vi "PressureGaugeWithSmallWindow.vi"(4 "Error In":errorcluster, 7 "Command":string) -> (0 "Error Out":errorcluster, 3 "Response":string)   [LabVIEW 2018]
uses:
  MOKO_LabViewLibrary/MokoLowLevel/MokoLowLovelControl/MLLC_Mode.ctl
  data/PressureGaugeInfo_1.ctl
panel:
  in  "Utility name":string="PRESSURESTORE"
  in  "Error Code":i32=5475
  in  "UtilitySettings":T2={"Permanent data"={"Информация об образце"={"Тип"="Манометр", "Владелец"="Компания \"MOKO\"", "Номер клейма"="111222", "Пределы допускаемой погрешности "=0.05, "Производственный № прибора"="111222333", "Наименование СИ"="Манометр"}, "Информация о поверке"={"Место проведения поверки"="Планета земля", "Поверку провел"="Johnny Respect", "Номер заказа"="1", "Номер рабочего места"="1", "ДД"=21.0, "ММ"="Январь", "ГГГГ"=2022.0, "№ протокола"="G-111111", "№ манометра"=5555.0}, "Характеристики манометра"={"Максимум шкалы"=10.0, "1-ая точка"=2.0, "Единица измерения"="МПа", "Цена деления"=2.0, "Класс точности"="0,4", "Минимум шкалы"=2.0, "Количество точек"=0.0}, "Условия поверки"={"Температура воздуха"=22.0, "Влажность воздуха"=60.0, "Давление"=750.0}, "Драйвер"="Simulation", "Поверяемая точка"=0.0}, "Saved Data"=variant(cluster{"Информация об образце":cluster{"Тип":string, "Владелец":string, "Номер клейма":string, "Пределы допускаемой погрешности ":dbl, "Производственный № прибора":string, "Наименование СИ":string}, "Информация о поверке":cluster{"Место проведения поверки":string, "Поверку провел":string, "Номер заказа":string, "Номер рабочего места":string, "ДД":dbl, "ММ":string, "ГГГГ":dbl, "№ протокола":string, "№ манометра":dbl}, "Характеристики манометра":cluster{"Максимум шкалы":dbl, "1-ая точка":dbl, "Единица измерения":string, "Цена деления":dbl, "Класс точности":string, "Минимум шкалы":dbl, "Количество точек":dbl}, "Условия поверки":cluster{"Температура воздуха":dbl, "Влажность воздуха":dbl, "Давление":dbl}, "Драйвер":string, "Поверяемая точка":dbl} {"Информация об образце"={"Тип"="Манометр", "Владелец"="Компания \"MOKO\"", "Номер клейма"="111222333", "Пределы допускаемой погрешности "=0.05, "Производственный № прибора"="111222333", "Наименование СИ"="Манометр"}, "Информация о поверке"={"Место проведения поверки"="Планета земля", "Поверку провел"="Johnny Respect", "Номер заказа"="1", "Номер рабочего места"="1", "ДД"=21.0, "ММ"="Январь", "ГГГГ"=2022.0, "№ протокола"="G-111111", "№ манометра"=1123123.0}, "Характеристики манометра"={"Максимум шкалы"=10.0, "1-ая точка"=2.0, "Единица измерения"="МПа", "Цена деления"=2.0, "Класс точности"="0,4", "Минимум шкалы"=2.0, "Количество точек"=0.0}, "Условия поверки"={"Температура воздуха"=22.0, "Влажность воздуха"=60.0, "Давление"=750.0}, "Драйвер"="Simulation", "Поверяемая точка"=0.0}), "waittime"=30000.0, "BAD"=0.0, "Defect"=FALSE}
  in  "Mode":T3=enum."Check"
  # "PressureGauge"
  # "Default Settings"
  # "Temporary data"
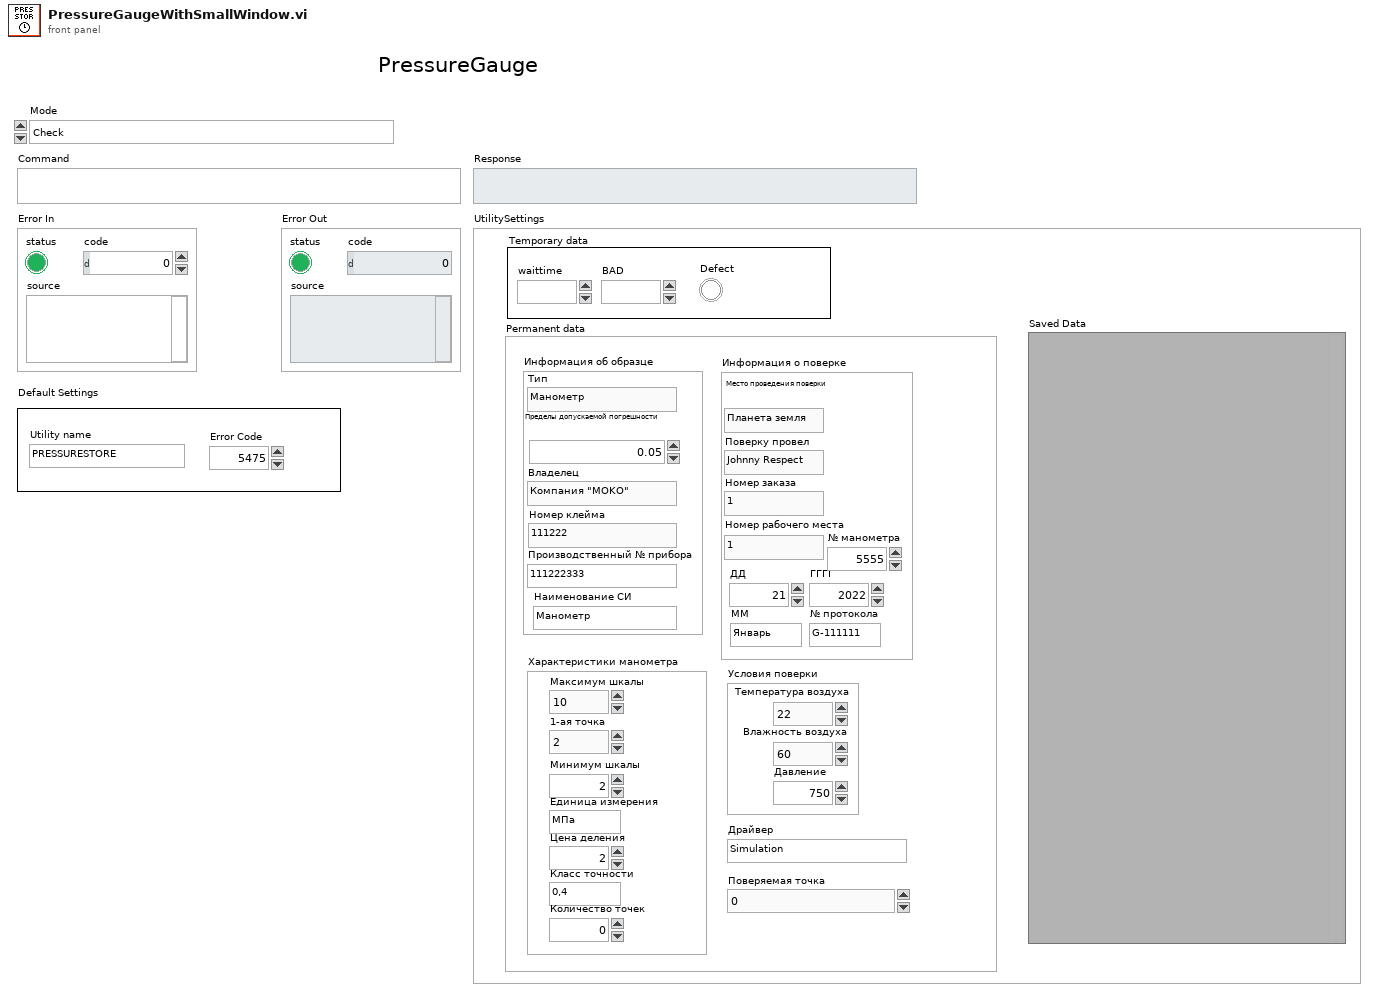
[diagram p1: front panel]
types:
  T1 = typedef "PressureGaugeInfo_1.ctl" = cluster{"Информация об образце":cluster{"Тип":string, "Владелец":string, "Номер клейма":string, "Пределы допускаемой погрешности ":dbl, "Производственный № прибора":string, "Наименование СИ":string}, "Информация о поверке":cluster{"Место проведения поверки":string, "Поверку провел":string, "Номер заказа":string, "Номер рабочего места":string, "ДД":dbl, "ММ":string, "ГГГГ":dbl, "№ протокола":string, "№ манометра":dbl}, "Характеристики манометра":cluster{"Максимум шкалы":dbl, "1-ая точка":dbl, "Единица измерения":string, "Цена деления":dbl, "Класс точности":string, "Минимум шкалы":dbl, "Количество точек":dbl}, "Условия поверки":cluster{"Температура воздуха":dbl, "Влажность воздуха":dbl, "Давление":dbl}, "Драйвер":string, "Поверяемая точка":dbl}
  T2 = cluster{"Permanent data":T1, "Saved Data":variant, "waittime":dbl, "BAD":dbl, "Defect":bool}
  T3 = typedef "MLLC_Mode.ctl" = enum16{"get", "set", "close", "Init", "Check"}
  T4 = typedef "MLLC_Error.ctl" = errorcluster
  T5 = typedef "PressureGaugeInfo.ctl" = cluster{"Информация об образце":cluster{"Тип":string, "Владелец":string, "Номер клейма":string, "Пределы допускаемой погрешности ":dbl, "Производственный № прибора":string, "Наименование СИ":string}, "Информация о поверке":cluster{"Место проведения поверки":string, "Поверку провел":string, "Номер заказа":string, "Номер рабочего места":string, "ДД":dbl, "ММ":string, "ГГГГ":dbl, "№ протокола":string, "№ манометра":dbl}, "Характеристики манометра":cluster{"Максимум шкалы":dbl, "1-ая точка":dbl, "Единица измерения":string, "Цена деления":dbl, "Класс точности":string, "Минимум шкалы":dbl, "Количество точек":dbl}, "Условия поверки":cluster{"Температура воздуха":dbl, "Влажность воздуха":dbl, "Давление":dbl}, "Драйвер":string, "Поверяемая точка":dbl}
  T6 = typedef "MLLC_Command.ctl" = string
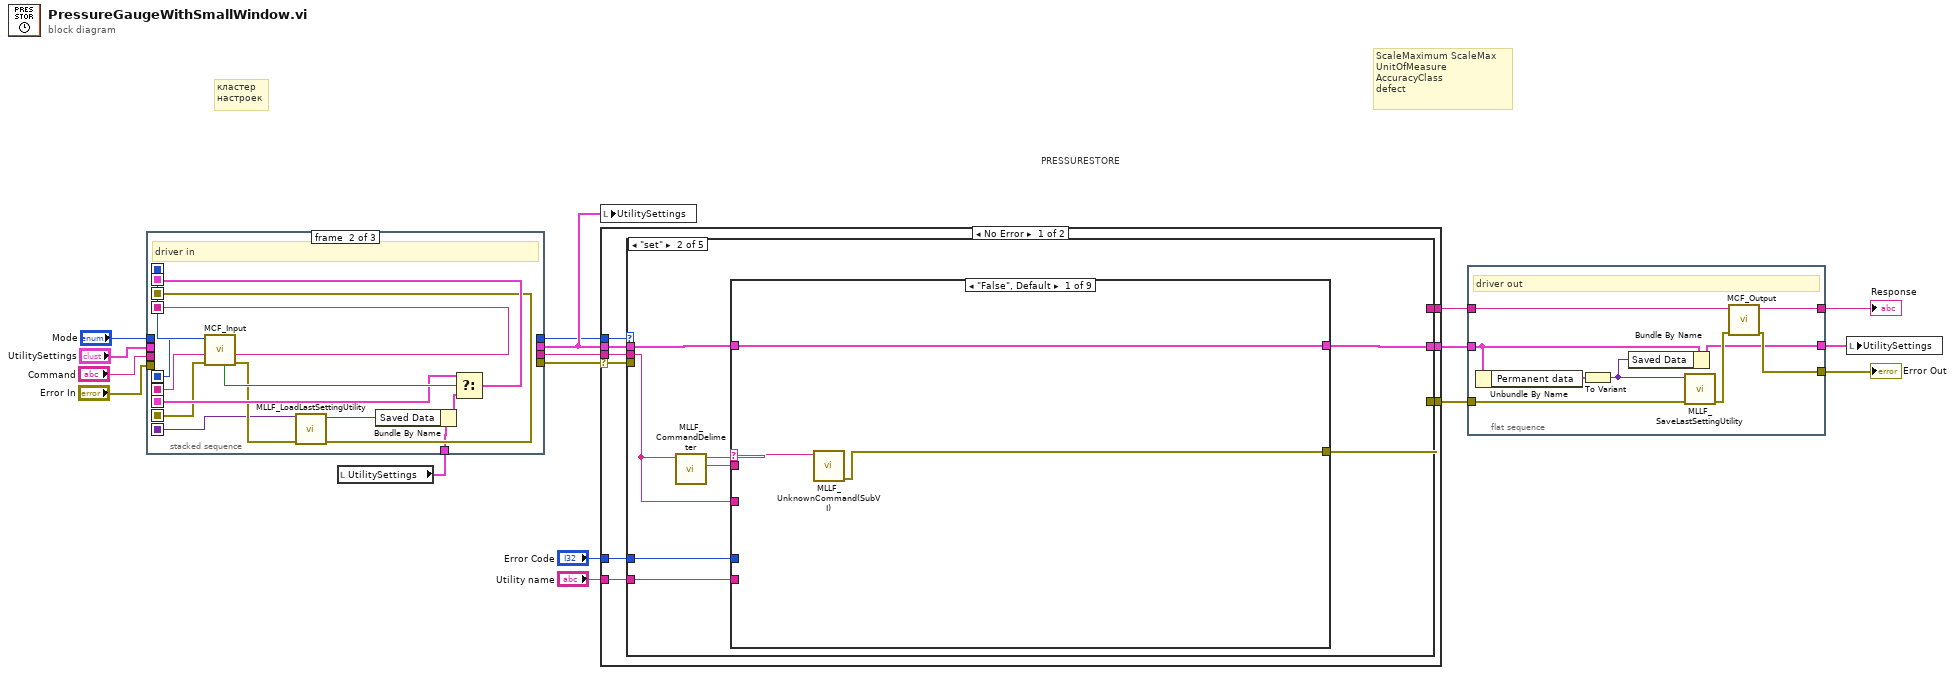
[diagram p0: block diagram]
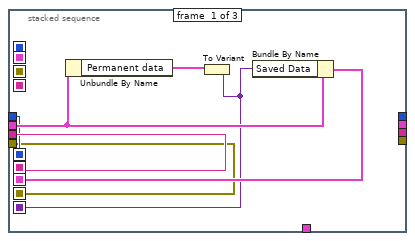
[diagram p2: hidden frame]
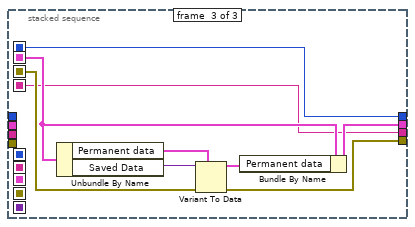
[diagram p3: hidden frame]
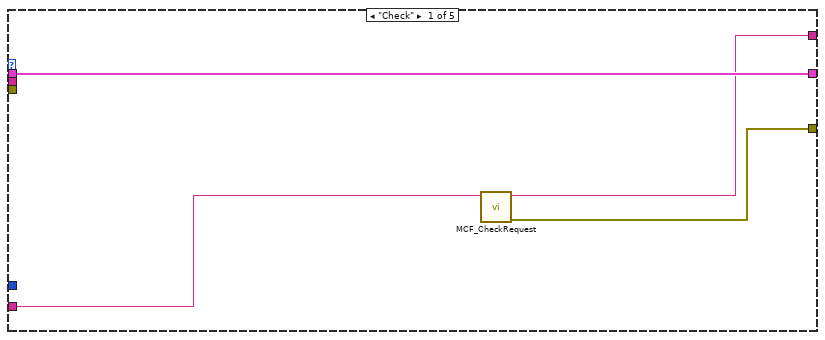
[diagram p4: hidden frame]
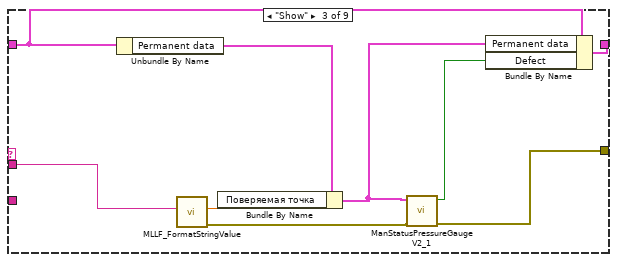
[diagram p6: hidden frame]
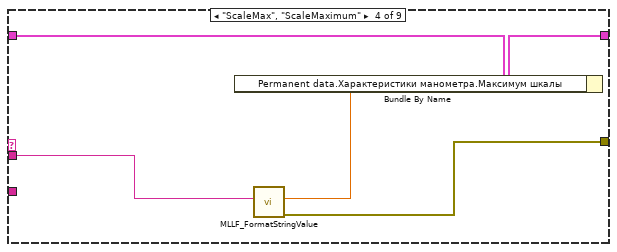
[diagram p7: hidden frame]
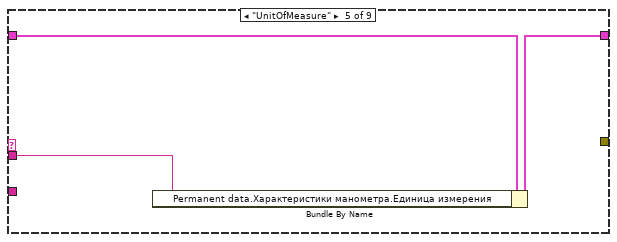
[diagram p8: hidden frame]
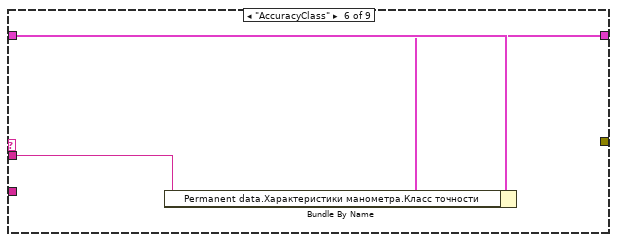
[diagram p9: hidden frame]
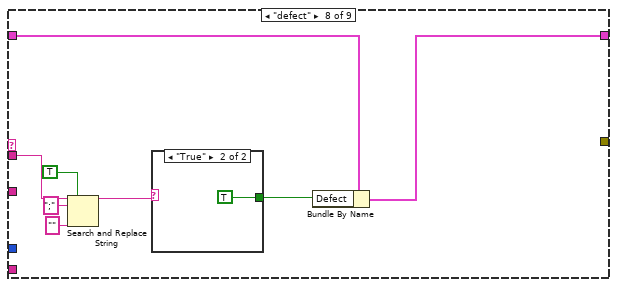
[diagram p11: hidden frame]
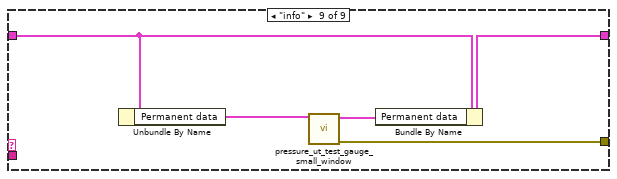
[diagram p13: hidden frame]
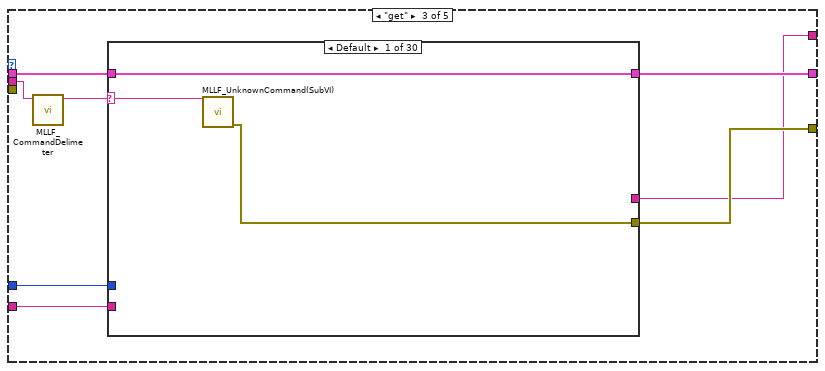
[diagram p14: hidden frame]
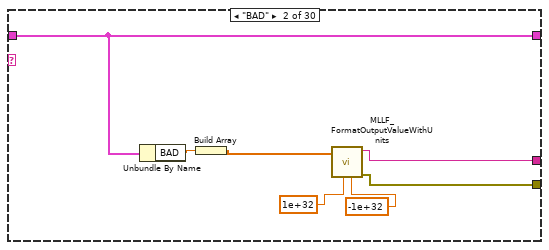
[diagram p15: hidden frame]
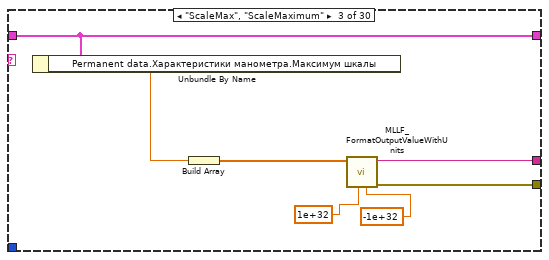
[diagram p16: hidden frame]
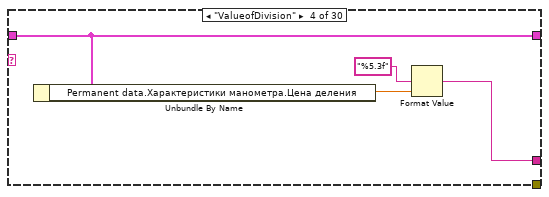
[diagram p17: hidden frame]
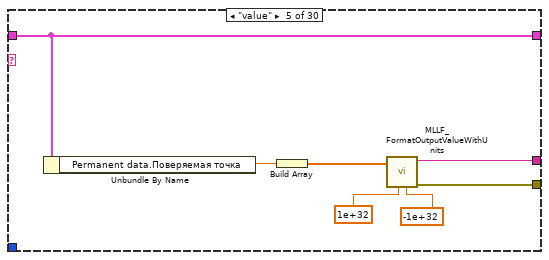
[diagram p18: hidden frame]
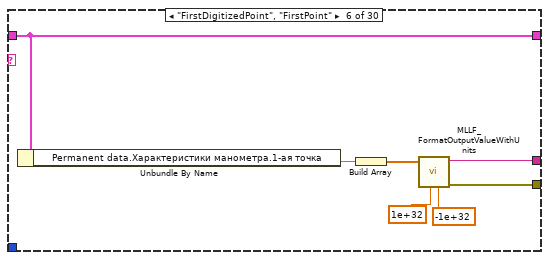
[diagram p19: hidden frame]
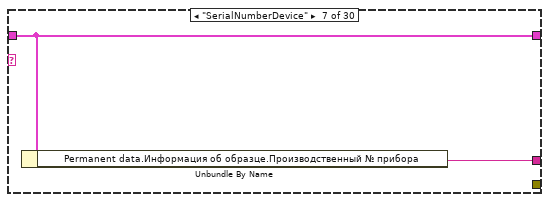
[diagram p20: hidden frame]
diagram:
  # "ScaleMaximum ScaleMax\nUnitOfMeasure\nAccuracyClass\ndefect"
  # "кластер\nнастроек"
  # "PRESSURESTORE"
  n1 = local read "UtilitySettings"() -> (w12:T2)
  n2 = stacked-sequence {
    seq-local: [w20 _ _] -> [_ w36 _]
    seq-local: [w19 _ _] -> [_ w37 _]
    seq-local: [w22 _ _] -> [_ w32 _]
    seq-local: [w18 _ _] -> [_ w31 _]
    seq-local: [w21 _ _] -> [_ w26 _]
    seq-local: [_ w27 _] -> [_ _ w43]
    seq-local: [_ w38 _] -> [_ _ w40]
    seq-local: [_ w35 _] -> [_ _ w39]
    seq-local: [_ w34 _] -> [_ _ w44]
    tunnel: "Command" -> [w20 _ _]
    tunnel: "Mode" -> [w19 _ _]
    tunnel: "Error In" -> [w18 _ _]
    tunnel: "UtilitySettings" -> [w23 _ _]
    tunnel: w12 -> [_ w25 _]
    tunnel: [_ _ w39] -> w8
    tunnel: [_ _ w42] -> w11
    tunnel: [_ _ w41] -> w10
    tunnel: [_ _ w40] -> w9
    frame #0 {
      n3 = Unbundle By Name(w23) -> ("Permanent data"=w24:T1)
      n4 = To Variant(anything=w24) -> (Variant=w21:variant)
      n5 = Bundle By Name(cluster=w23, "Saved Data"=w21) -> (w22:T2)
    }
    frame #1 {
      # "driver in"
      n6 = call "MCF_Input.vi"("error in (no error)"=w31, "Command"=w36, "Mode"=w37) -> ("error out"=w30:errorcluster, "Command out"=w35:string, "Mode out"=w38:T3, "Boolean"=w33:bool)  [unwired: 5 in]
      n7 = call "MLLF_LoadLastSettingUtility.vi"("Error In"=w30, "Save data in"=w26) -> ("Error Out"=w27:errorcluster, "Save data out"=w29:variant)  [unwired: 8 in]
      n8 = Bundle By Name(cluster=w25, "Saved Data"=w29) -> (w28:T2)
      n9 = Select(t=w32, s=w33, f=w28) -> (s? t:f=w34:T2)
    }
    frame #2 {
      n10 = Unbundle By Name(w44) -> ("Permanent data"=w45:T1, "Saved Data"=w47:variant)
      n11 = Variant To Data(error in=w43, type=w45, Variant=w47) -> (data=w46:T1, error out=w41:errorcluster)
      n12 = Bundle By Name(cluster=w44, "Permanent data"=w46) -> (w42:T2)
    }
  }
  n13 = local write "UtilitySettings"(w11) -> ()
  n14 = case shown="No Error" w10 {
    selector: w10 -> [w52 w234]
    tunnel: [w54 w234] -> w16
    tunnel: w9 -> [w56 _]
    tunnel: [w55 _] -> w14
    tunnel: w8 -> [w53 _]
    tunnel: w11 -> [w49 w233]
    tunnel: "Error Code" -> [w51 _]
    tunnel: "Utility name" -> [w50 _]
    tunnel: [w48 w233] -> w15
    frame No Error {
      n15 = case shown="\"set\"" w56 {
        tunnel: [w58 _ w108 _ _] -> w55
        tunnel: [w57 w68 w109 _ _] -> w54
        tunnel: w53 -> [_ w63 w115 _ _]
        tunnel: w52 -> [_ _ _ _ _]
        tunnel: w51 -> [_ w67 w112 _ _]
        tunnel: w50 -> [w59 w64 w111 _ _]
        tunnel: w49 -> [w60 w66 w114 w231 w232]
        tunnel: [w60 w65 w113 w231 w232] -> w48
        frame "Check" {
          n16 = call "MCF_CheckRequest.vi"("Driver Name"=w59) -> ("Error Out"=w57:errorcluster, "Output String"=w58:string)  [unwired: 9 in]
        }
        frame "set" {
          n17 = call "MLLF_CommandDelimeter.vi"("command with param"=w63) -> ("param 1"=w61:string, "command"=w62:string)  [unwired: 7 in, 2 out]
          n18 = case shown="\"False\", Default" w62 {
            selector: w62 -> [w70 _ _ _ _ _ _ _ _]
            tunnel: w61 -> [_ _ w78 w82 w88 w92 _ w99 _]
            tunnel: w63 -> [_ _ _ _ _ _ _ _ _]
            tunnel: [w69 _ w75 w86 _ _ _ _ w107] -> w68
            tunnel: w67 -> [_ _ _ _ _ _ _ _ _]
            tunnel: w66 -> [w71 w72 w80 w84 w89 w91 w93 w101 w106]
            tunnel: [w71 w72 w79 w83 w87 w90 w93 w100 w105] -> w65
            tunnel: w64 -> [_ _ _ _ _ _ _ _ _]
            frame "False", Default {
              n19 = call "MLLF_UnknownCommand(SubVI).vi"("Unknown command"=w70) -> ("error out"=w69:errorcluster)  [unwired: 10 in]
            }
            frame "<----MAIN FUNCTIONS---->" {
            }
            frame "Show" {
              n20 = Unbundle By Name(w80) -> ("Permanent data"=w74:T1)
              n21 = call "MLLF_FormatStringValue.vi"("String Value"=w78) -> ("error out"=w77:T4, "number"=w81:dbl)  [unwired: 8 in, 1 out]
              n22 = Bundle By Name(cluster=w74, "Поверяемая точка"=w81) -> (w73:T1)
              n23 = call "ManStatusPressureGaugeV2_1.vi"("Error In"=w77, "Show in"=w73) -> ("Error Out"=w75:errorcluster, "defect"=w76:bool)  [unwired: 8 in]
              n24 = Bundle By Name(cluster=w80, "Permanent data"=w73, "Defect"=w76) -> (w79:T2)
            }
            frame "ScaleMax", "ScaleMaximum" {
              n25 = call "MLLF_FormatStringValue.vi"("String Value"=w82) -> ("error out"=w86:T4, "number"=w85:dbl)  [unwired: 8 in, 1 out]
              n26 = Bundle By Name(cluster=w84, "Permanent data.Характеристики манометра.Максимум шкалы"=w85) -> (w83:T2)
            }
            frame "UnitOfMeasure" {
              n27 = Bundle By Name(cluster=w89, "Permanent data.Характеристики манометра.Единица измерения"=w88) -> (w87:T2)
            }
            frame "AccuracyClass" {
              n28 = Bundle By Name(cluster=w91, "Permanent data.Характеристики манометра.Класс точности"=w92) -> (w90:T2)
            }
            frame "---------ADDITIONAL---------" {
            }
            frame "defect" {
              n29 = Search and Replace String(replace all?=TRUE ("replace all? (F)"), input string=w99, search string=";", replace string="" ("replace string (\"\")")) -> (result string=w95:string)  [unwired: 4 in, 3 out]
              n30 = case shown="\"True\"" w95 {
                tunnel: [_ TRUE] -> w94
                frame "False", Default {
                }
                frame "True" {
                }
              }
              n31 = Bundle By Name(cluster=w101, "Defect"=w94) -> (w100:T2)
            }
            frame "info" {
              n32 = Unbundle By Name(w106) -> ("Permanent data"=w103:T1)
              n33 = call "pressure_ut_test_gauge_small_window.vi"("Manometr in"=w103) -> ("Error Out"=w107:errorcluster, "Manometr out"=w104:T5)  [unwired: 9 in]
              n34 = Bundle By Name(cluster=w106, "Permanent data"=w104) -> (w105:T2)
            }
          }
        }
        frame "get" {
          n35 = call "MLLF_CommandDelimeter.vi"("command with param"=w115) -> ("command"=w110:string)  [unwired: 7 in, 3 out]
          n36 = case shown="Default" w110 {
            selector: w110 -> [w117 _ _ _ _ _ _ _ _ _ _ _ _ _ _ _ _ _ _ _ _ _ _ _ _ _ _ _ _ _]
            tunnel: w112 -> [_ _ _ _ _ _ _ _ _ _ _ _ _ _ _ _ _ _ _ _ _ _ _ _ _ _ _ _ _ _]
            tunnel: [w118 w125 w132 w136 w143 w150 w152 w154 w161 w168 w170 w172 w174 w181 w183 w186 w188 w191 w193 w197 w199 w203 w205 w209 w211 w215 w219 w223 w225 w230] -> w113
            tunnel: w114 -> [w118 w125 w132 w136 w143 w150 w152 w154 w161 w168 w170 w172 w174 w181 w183 w186 w188 w191 w193 w197 w199 w203 w205 w209 w211 w215 w219 w223 w225 w230]
            tunnel: w111 -> [_ _ _ _ _ _ _ _ _ _ _ _ _ _ _ _ _ _ _ _ _ _ _ _ _ _ _ _ _ _]
            tunnel: [w116 w120 w126 _ w138 w145 _ _ w155 w162 _ _ _ w175 _ _ _ _ _ _ _ _ _ _ _ _ _ _ _ _] -> w109
            tunnel: [_ w121 w127 w133 w137 w146 w151 w153 w156 w163 w169 w171 w173 w176 w182 w184 w187 w189 w192 w194 w198 w200 w204 w206 w210 w212 w216 w220 w224 w226] -> w108
            frame Default {
              n37 = call "MLLF_UnknownCommand(SubVI).vi"("Unknown command"=w117) -> ("error out"=w116:errorcluster)  [unwired: 10 in]
            }
            frame "BAD" {
              n38 = Unbundle By Name(w125) -> ("BAD"=w124:dbl)
              n39 = Build Array(w124) -> (w122:dbl[])
              n40 = call "MLLF_FormatOutputValueWithUnits.vi"("Lower limit"=-1e+32, "Upper limit"=1e+32, "ValuesIn"=w122) -> ("error out"=w120:T4, "Result string"=w121:T6)  [unwired: 7 in]
            }
            frame "ScaleMax", "ScaleMaximum" {
              n41 = Unbundle By Name(w132) -> ("Permanent data.Характеристики манометра.Максимум шкалы"=w131:dbl)
              n42 = Build Array(w131) -> (w128:dbl[])
              n43 = call "MLLF_FormatOutputValueWithUnits.vi"("Lower limit"=-1e+32, "Upper limit"=1e+32, "ValuesIn"=w128) -> ("error out"=w126:T4, "Result string"=w127:T6)  [unwired: 7 in]
            }
            frame "ValueofDivision" {
              n44 = Unbundle By Name(w136) -> ("Permanent data.Характеристики манометра.Цена деления"=w134:dbl)
              n45 = Format Value(format string="%5.3f", value (0)=w134) -> (output string=w133:string)  [unwired: 1 in]
            }
            frame "value" {
              n46 = Unbundle By Name(w143) -> ("Permanent data.Поверяемая точка"=w142:dbl)
              n47 = Build Array(w142) -> (w139:dbl[])
              n48 = call "MLLF_FormatOutputValueWithUnits.vi"("Lower limit"=-1e+32, "Upper limit"=1e+32, "ValuesIn"=w139) -> ("error out"=w138:T4, "Result string"=w137:T6)  [unwired: 7 in]
            }
            frame "FirstDigitizedPoint", "FirstPoint" {
              n49 = Unbundle By Name(w150) -> ("Permanent data.Характеристики манометра.1-ая точка"=w149:dbl)
              n50 = Build Array(w149) -> (w147:dbl[])
              n51 = call "MLLF_FormatOutputValueWithUnits.vi"("Lower limit"=-1e+32, "Upper limit"=1e+32, "ValuesIn"=w147) -> ("error out"=w145:T4, "Result string"=w146:T6)  [unwired: 7 in]
            }
            frame "SerialNumberDevice" {
              n52 = Unbundle By Name(w152) -> ("Permanent data.Информация об образце.Производственный № прибора"=w151:string)
            }
            frame "NameMI" {
              n53 = Unbundle By Name(w154) -> ("Permanent data.Информация об образце.Наименование СИ"=w153:string)
            }
            frame "NumOfPoints" {
              n54 = Unbundle By Name(w161) -> ("Permanent data.Характеристики манометра.Количество точек"=w160:dbl)
              n55 = Build Array(w160) -> (w157:dbl[])
              n56 = call "MLLF_FormatOutputValueWithUnits.vi"("Lower limit"=-1e+32, "Upper limit"=1e+32, "ValuesIn"=w157) -> ("error out"=w155:T4, "Result string"=w156:T6)  [unwired: 7 in]
            }
            frame "ScaleMin" {
              n57 = Unbundle By Name(w168) -> ("Permanent data.Характеристики манометра.Минимум шкалы"=w167:dbl)
              n58 = Build Array(w167) -> (w164:dbl[])
              n59 = call "MLLF_FormatOutputValueWithUnits.vi"("Lower limit"=-1e+32, "Upper limit"=1e+32, "ValuesIn"=w164) -> ("error out"=w162:T4, "Result string"=w163:T6)  [unwired: 7 in]
            }
            frame "UnitOfMeasure" {
              n60 = Unbundle By Name(w170) -> ("Permanent data.Характеристики манометра.Единица измерения"=w169:string)
            }
            frame "AccuracyClass" {
              n61 = Unbundle By Name(w172) -> ("Permanent data.Характеристики манометра.Класс точности"=w171:string)
            }
            frame "TypeofUnit" {
              n62 = Unbundle By Name(w174) -> ("Permanent data.Информация об образце.Тип"=w173:string)
            }
            frame "PermissibleError" {
              (unwired) "%5.4f" ("format string")
              n63 = Unbundle By Name(w181) -> ("Permanent data.Информация об образце.Пределы допускаемой погрешности"=w180:dbl)
              n64 = Build Array(w180) -> (w177:dbl[])
              n65 = call "MLLF_FormatOutputValueWithUnits.vi"("Lower limit"=-1e+32, "Upper limit"=1e+32, "ValuesIn"=w177) -> ("error out"=w175:T4, "Result string"=w176:T6)  [unwired: 7 in]
            }
            frame "StampNumber" {
              n66 = Unbundle By Name(w183) -> ("Permanent data.Информация об образце.Номер клейма"=w182:string)
            }
            frame "Owner" {
              n67 = Unbundle By Name(w186) -> ("Permanent data.Информация об образце.Владелец"=w185:string)
              n68 = call "MLLF_ReplaceTwoQuotesWithOne.vi"("String in"=w185) -> ("Result string"=w184:string)  [unwired: 7 in, 3 out]
            }
            frame "Verifier" {
              n69 = Unbundle By Name(w188) -> ("Permanent data.Информация о поверке.Поверку провел"=w187:string)
            }
            frame "VerificationLocation" {
              n70 = Unbundle By Name(w191) -> ("Permanent data.Информация о поверке.Место проведения поверки"=w190:string)
              n71 = call "MLLF_ReplaceTwoQuotesWithOne.vi"("String in"=w190) -> ("Result string"=w189:string)  [unwired: 7 in, 3 out]
            }
            frame "WorkplaceNumber" {
              n72 = Unbundle By Name(w193) -> ("Permanent data.Информация о поверке.Номер рабочего места"=w192:string)
            }
            frame "UnitNumber" {
              n73 = Unbundle By Name(w197) -> ("Permanent data.Информация о поверке.№ манометра"=w195:dbl)
              n74 = Format Value(format string="%5.1f", value (0)=w195) -> (output string=w194:string)  [unwired: 1 in]
            }
            frame "OrderNumber" {
              n75 = Unbundle By Name(w199) -> ("Permanent data.Информация о поверке.Номер заказа"=w198:string)
            }
            frame "Day" {
              n76 = Unbundle By Name(w203) -> ("Permanent data.Информация о поверке.ДД"=w201:dbl)
              n77 = Format Value(format string="%#g", value (0)=w201) -> (output string=w200:string)  [unwired: 1 in]
            }
            frame "Month" {
              n78 = Unbundle By Name(w205) -> ("Permanent data.Информация о поверке.ММ"=w204:string)
            }
            frame "Year" {
              n79 = Unbundle By Name(w209) -> ("Permanent data.Информация о поверке.ГГГГ"=w207:dbl)
              n80 = Format Value(format string="%#g", value (0)=w207) -> (output string=w206:string)  [unwired: 1 in]
            }
            frame "ProtocolNumber" {
              n81 = Unbundle By Name(w211) -> ("Permanent data.Информация о поверке.№ протокола"=w210:string)
            }
            frame "Temperature" {
              n82 = Unbundle By Name(w215) -> ("Permanent data.Условия поверки.Температура воздуха"=w214:dbl)
              n83 = Format Value(format string="%5.1f", value (0)=w214) -> (output string=w212:string)  [unwired: 1 in]
            }
            frame "AmbientPressure" {
              n84 = Unbundle By Name(w219) -> ("Permanent data.Условия поверки.Давление"=w217:dbl)
              n85 = Format Value(format string="%5.1f", value (0)=w217) -> (output string=w216:string)  [unwired: 1 in]
            }
            frame "Humidity" {
              n86 = Unbundle By Name(w223) -> ("Permanent data.Условия поверки.Влажность воздуха"=w221:dbl)
              n87 = Format Value(format string="%5.1f", value (0)=w221) -> (output string=w220:string)  [unwired: 1 in]
            }
            frame "Driver" {
              n88 = Unbundle By Name(w225) -> ("Permanent data.Драйвер"=w224:string)
            }
            frame "defect" {
              n89 = Unbundle By Name(w230) -> ("Defect"=w227:bool)
              n90 = Select(t="True" ("string"), s=w227, f="False" ("string")) -> (s? t:f=w226:string)
            }
          }
        }
        frame "close" {
        }
        frame "Init" {
        }
      }
    }
    frame Error {
    }
  }
  n91 = flat-sequence {
    tunnel: [w243] -> w6
    tunnel: [w242] -> w4
    tunnel: w14 -> [w241]
    tunnel: w16 -> [w240]
    tunnel: w15 -> [w236]
    tunnel: [w238] -> w13
    frame #0 {
      # "driver out"
      n92 = Unbundle By Name(w236) -> ("Permanent data"=w235:T1)
      n93 = To Variant(anything=w235) -> (Variant=w237:variant)
      n94 = Bundle By Name(cluster=w236, "Saved Data"=w237) -> (w238:T2)
      n95 = call "MLLF_SaveLastSettingUtility.vi"("error in"=w240, "Saved Data"=w237) -> ("error out"=w239:T4)  [unwired: 8 in, 1 out]
      n96 = call "MCF_Output.vi"("Error In"=w239, "Input"=w241) -> ("Error Out"=w242:errorcluster, "Output"=w243:string)  [unwired: 8 in]
    }
  }
  n97 = local write "UtilitySettings"(w13) -> ()
  "Response" <- w6
  "Error Out" <- w4
